vi "6131demo.vi"() -> ()   [LabVIEW 2012]
panel:
  in  "停止":bool
  out "数组":dbl[](array[numeric])
  out "U8":u8[](array[numeric])
  out "*(类型 *) &x":u32 format="%.0x"
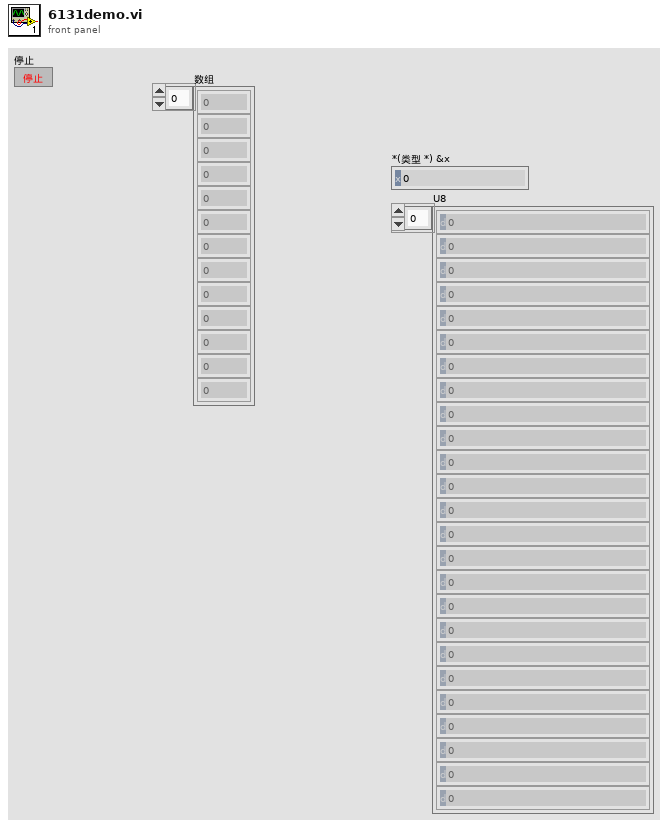
[diagram p1: front panel]
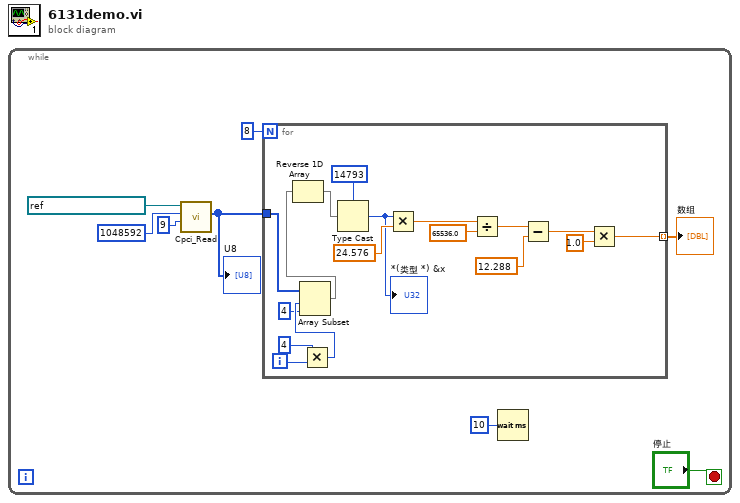
[diagram p0: block diagram]
diagram:
  n1 = while {
    stop <- "停止" stop-if-true
    n2 = call "Cpci_Read.vi"("u32_len"=9, "基地址"=u32 1048592, "VISA资源名称"=refnum<visa-resource-name> "PXI1::14::INSTR") -> ("U8"=w4:u8[])  [unwired: 6 in, 2 out]
    "U8" <- w4
    n3 = for {
      N: 8 -> [_]
      tunnel: w4 -> [w16]
      tunnel: [w9] -> w3 mode=indexing
      i -> [w15]
      n4 = Multiply(x=4, y=w15) -> (x*y=w13:i32)
      n5 = Array Subset(array=w16, index=w13, length=4 ("长度")) -> (w11:u8[])
      n6 = Reverse 1D Array(array=w11) -> (reversed array=w10:u8[])
      n7 = Type Cast(type=u32 14793 ("x"), x=w10) -> (*(type *) &x=w18:u32)
      "*(类型 *) &x" <- w18
      n8 = Multiply(x=w18, y=24.576) -> (x*y=w24:dbl)
      n9 = Divide(x=w24, y=65536.0) -> (x/y=w22:dbl)
      n10 = Subtract(x=w22, y=12.288) -> (x-y=w20:dbl)
      n11 = Multiply(x=w20, y=1.0) -> (x*y=w9:dbl)
    }
    "数组" <- w3
    n12 = Wait (ms)(milliseconds to wait=u32 10 ("等待时间（毫秒）")) -> ()  [unwired: 1 out]
  }
